vi "EPTxRTadd_ontest5.vi"(9 "Falling":sgl, 10 "Rising":sgl, 11 "switch":bool) -> (1 "FallingCAD":fxp<+,18,11>, 2 "RisingCAD":fxp<+,18,11>, 3 "Switch_out":bool)   [LabVIEW 2020]
uses:
  <vilib>/Powertrain Controls/Device Drivers/Engine Position Tracking/EPTx/RevA/RT/Controls/EPTxAAPControl.ctl
  <vilib>/Powertrain Controls/Device Drivers/Engine Position Tracking/EPTx/RevA/RT/EPTx - RevA - RT.lvlib
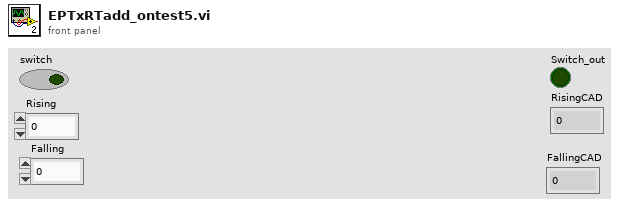
[diagram p1: front panel]
types:
  T1 = typedef "EPTx - RevA - RT.lvlib/EPTxAAPControl.ctl" = cluster{"Enable":bool, "Rising_[DBTDC]":sgl, "Falling_[DBTDC]":sgl}
  T2 = typedef "EPTx - RevA - FPGA.lvlib/EPTxAAPControl.ctl" = cluster{"Enable":bool, "RisingCAD":fxp<+,18,11>, "FallingCAD":fxp<+,18,11>}
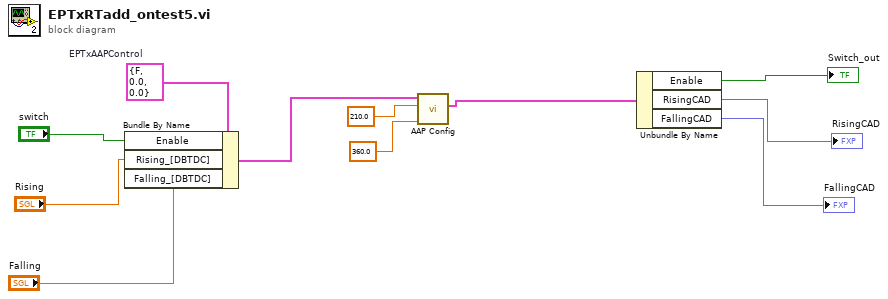
[diagram p0: block diagram]
diagram:
  w9 = T1 {"Enable"=FALSE, "Rising_[DBTDC]"=0.0, "Falling_[DBTDC]"=0.0}  # EPTxAAPControl
  n1 = Bundle By Name(cluster=w9, "Enable"="switch", "Rising_[DBTDC]"="Rising", "Falling_[DBTDC]"="Falling") -> (w8:T1)
  n2 = call <vilib>:"AAP Config.vi"("Max CAD"=sgl 360.0, "Cylinder TDC [Absolute CAD]"=sgl 210.0, "EPTxAAPControl"=w8) -> ("EPTxAAPControl"=w7:T2)  [unwired: 8 in]
  n3 = Unbundle By Name(w7) -> ("Enable"=→"Switch_out":bool, "RisingCAD"=→"RisingCAD":fxp<+,18,11>, "FallingCAD"=→"FallingCAD":fxp<+,18,11>)
